vi "draw_overlay.vi"(8 "error in (no error)":errorcluster, 11 "ScanModeDL091001Scaffold in":refnum<class "ImagingModeDL091001Scaffold.lvclass">) -> (0 "error out":errorcluster, 3 "ScanModeDL091001Scaffold out":refnum<class "ImagingModeDL091001Scaffold.lvclass">)   [LabVIEW 2010]
uses:
  Adapter/GenericAdapter/GenericAdapter/GenericAdapter.lvclass
  ImagingModeDL091001Scaffold.lvclass
  Trajectory/GenericTrajectory/GenericTrajectory/GenericTrajectory.lvclass
  common/classes/GenericComponent/GenericComponent/GenericComponent.lvclass
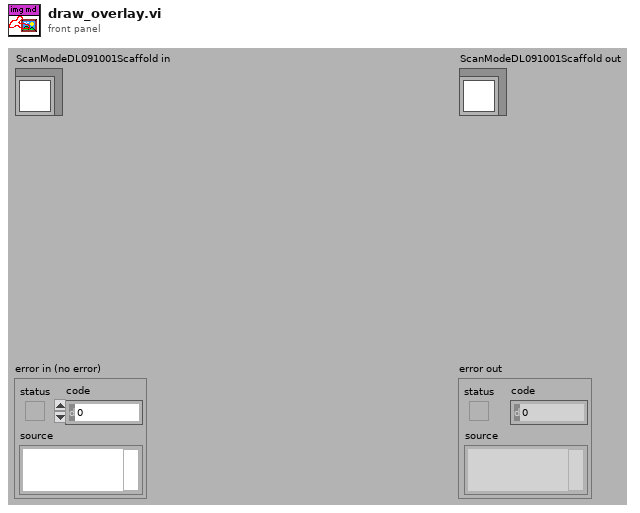
[diagram p1: front panel]
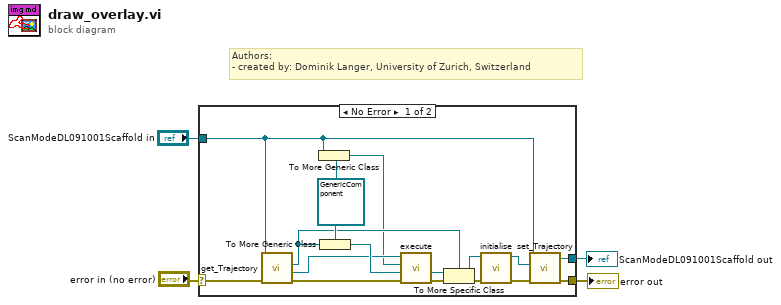
[diagram p0: block diagram]
diagram:
  # "Authors: \n- created by: Dominik Langer, University of Zurich, Switzerland"
  n1 = case shown="No Error" "error in (no error)" {
    selector: "error in (no error)" -> [w20 w22]
    tunnel: [w6 w22] -> w3
    tunnel: [w5 w21] -> w1
    tunnel: "ScanModeDL091001Scaffold in" -> [w11 w21]
    frame No Error {
      w19 = refnum<class "GenericComponent.lvclass"> refnum ("GenericComponent.lvclass")
      n2 = call-dynamic "get_Trajectory.vi"("error in (no error)"=w20, "ScanModeDL090923Scaffold in"=w11) -> ("error out"=w17:errorcluster, "Trajectory adapter"=w14:refnum<class "GenericAdapter.lvclass">, "Trajectory"=w13:refnum<class "GenericTrajectory.lvclass">)  [unwired: 2 in, 5 out]
      n3 = To More Generic Class(target class=w19, reference=w11) -> (generic class reference=w12:refnum<class "GenericComponent.lvclass">)
      n4 = To More Generic Class(target class=w19, reference=w13) -> (generic class reference=w18:refnum<class "GenericComponent.lvclass">)
      n5 = call-dynamic "execute.vi"("error in (no error)"=w17, "B in"=w18, "A in"=w12, "GenericAdapter in"=w14) -> ("error out"=w16:errorcluster, "B out"=w15:refnum<class "GenericComponent.lvclass">)  [unwired: 4 in, 2 out]
      n6 = To More Specific Class(target class=w13, reference=w15, error in=w16) -> (specific class reference=w9:refnum<class "GenericTrajectory.lvclass">, error out=w10:errorcluster)
      n7 = call-dynamic "initialise.vi"("error in (no error)"=w10, "GenericPlugin in"=w9) -> ("error out"=w7:errorcluster, "GenericPlugin out"=w8:refnum<class "GenericTrajectory.lvclass">)  [unwired: 8 in]
      n8 = call-dynamic "set_Trajectory.vi"("error in (no error)"=w7, "GenericTrajectory.lvclass"=w8, "ScanModeDL090923Scaffold in"=w11) -> ("error out"=w6:errorcluster, "ScanModeDL090923Scaffold out"=w5:refnum<class "ImagingModeDL091001Scaffold.lvclass">)  [unwired: 7 in]
    }
    frame Error {
    }
  }
  "error out" <- w3
  "ScanModeDL091001Scaffold out" <- w1
